vi "Simple Bluetooth - Client.vi"() -> ()   [LabVIEW 2023]
doc: "Demonstrates how to open a connection to a specified Bluetooth server and channel, read the data being sent to the channel, and display the data on a chart. This VI is designed to stop if the Bluetooth connection is terminated."
panel:
  in  "Server Closed":string="The server VI closed the connection."
  out "Waveform Graph":dbl[](graph)
  in  "Channel":u16
  in  "Address":string
  in  "Stop":bool
  # "Overview: Demonstrates the use of the Bluetooth functions to connect to a Bluetooth server VI and receive data.\nRequirements: Bluetooth-enabled computer\nInstructions:\n1. Ensure Simple Bluetooth - Server.vi is already running.\n2. Specify the same Address and Channel displayed on the front panel of Simple Bluetooth - Server.vi.\n3. Run the VI.\n4. Click Stop to stop the VI. Note that if you stop the server VI, this VI will stop automatically."
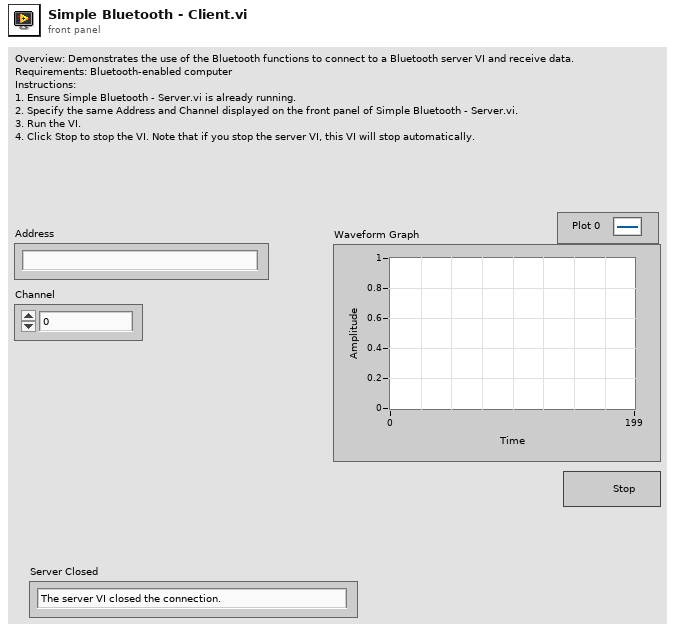
[diagram p1: front panel]
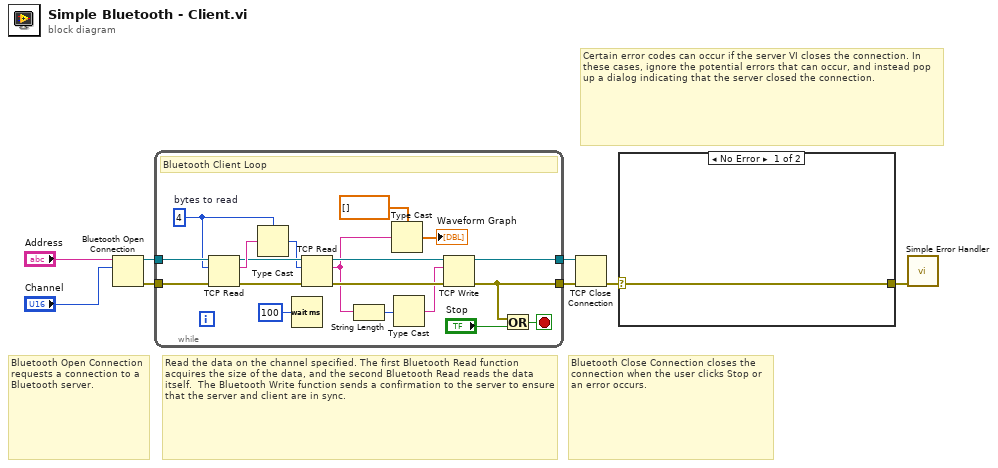
[diagram p0: block diagram]
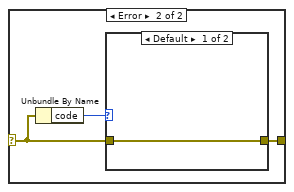
[diagram p2: hidden frame]
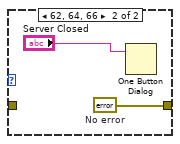
[diagram p3: hidden frame]
diagram:
  # "Certain error codes can occur if the server VI closes the connection. In these cases, ignore the potential errors that can occur, and instead pop up a dialog indicating that the server closed the connection."
  # "Bluetooth Close Connection closes the connection when the user clicks Stop or an error occurs."
  # "Read the data on the channel specified. The first Bluetooth Read function acquires the size of the data, and the second Bluetooth Read reads the data itself.  The Bluetooth Write function sends a confirmation to the server to ensure that the server and client are in sync."
  # "Bluetooth Open Connection requests a connection to a Bluetooth server."
  n1 = Bluetooth Open Connection(10:"Channel", 11:"Address") -> (0:w5:errorcluster, 3:w6:refnum<k31>)  [unwired: 3 in]
  n2 = while {
    tunnel: w5 -> [w22]
    tunnel: w6 -> [w23]
    tunnel: [w15] -> w7
    tunnel: [w10] -> w8
    stop <- w20 stop-if-true
    w9 = 4  # bytes to read
    # "Bluetooth Client Loop"
    n3 = TCP Read(connection ID=w23, bytes to read=w9, error in (no error)=w22) -> (connection ID out=w26:refnum<k31>, data out=w27:string, error out=w25:errorcluster)  [unwired: 2 in]
    n4 = Type Cast(type=w9, x=w27) -> (*(type *) &x=w24:i32)
    n5 = Wait (ms)(milliseconds to wait=u32 100) -> ()  [unwired: 1 out]
    n6 = TCP Read(connection ID=w26, bytes to read=w24, error in (no error)=w25) -> (connection ID out=w16:refnum<k31>, data out=w13:string, error out=w14:errorcluster)  [unwired: 2 in]
    n7 = String Length(string=w13) -> (length=w12:i32)
    n8 = Type Cast(type=dbl[] [] ("chart"), x=w13) -> (*(type *) &x=→"Waveform Graph":dbl[])
    n9 = Type Cast(x=w12) -> (*(type *) &x=w11:string)  [unwired: 1 in]
    n10 = TCP Write(connection ID=w16, data in=w11, error in (no error)=w14) -> (connection ID out=w15:refnum<k31>, error out=w10:errorcluster)  [unwired: 1 in, 1 out]
    n11 = Or(x=w10, y="Stop") -> (x .or. y?=w20:bool)
  }
  n12 = TCP Close Connection(connection ID=w7, error in (no error)=w8) -> (error out=w2:errorcluster)  [unwired: 1 in, 1 out]
  n13 = case shown="No Error" w2 {
    selector: w2 -> [w28 w30]
    tunnel: [w28 w29] -> w1
    frame No Error {
    }
    frame Error {
      n14 = Unbundle By Name(w30) -> ("code"=w31:i32)
      n15 = case shown="Default" w31 {
        tunnel: w30 -> [w32 _]
        tunnel: [w32 w34] -> w29
        frame Default {
        }
        frame 62, 64, 66 {
          w34 = errorcluster {"status"=FALSE, "code"=0, "source"=""}  # No error
          n16 = One Button Dialog(message="Server Closed") -> ()  [unwired: 1 in, 1 out]
        }
      }
    }
  }
  n17 = call <vilib>:"Simple Error Handler.vi"("error in (no error)"=w1) -> ()  [unwired: 4 in, 5 out]
